vi "Render Inverted Section with Empty Map Object Array.vi"(8 "Error In":errorcluster) -> (0 "Error Out":errorcluster)   [LabVIEW 2018, in "Tests.lvlib" / "Render.lvlib"]
uses:
  Render.lvlib
  <vilib>/addons/_JKI Toolkits/Caraya/classes/Test/Test.lvclass
  <vilib>/addons/_JKI Toolkits/Caraya/classes/Assert/Assert.lvclass
  src/Toolkit/Data/Array/Array.lvclass
  src/Toolkit/Low-Level/Renderer/Abstract/Render to String.vi
  src/Toolkit/Low-Level/Support/Lex String.vi
  src/Toolkit/Data/Array/Support/From Data.vi
  src/Toolkit/Data/Pair/Pair.lvclass
  src/Toolkit/Data/Pair/Support/From Datum.vi
  src/Toolkit/Data/Map/Map.lvclass
  src/Toolkit/Low-Level/Context/Compiler.lvclass
  D:/Users/cfield/Code/Field R&D Services/Labstache/src/Toolkit/Data/Datum/Datum.lvclass
  src/Toolkit/Low-Level/Nodes/Root/Root.lvclass
  D:/Users/cfield/Code/Field R&D Services/Labstache/src/Toolkit/Low-Level/Nodes/NonTerminal/NonTerminal.lvclass
  D:/Users/cfield/Code/Field R&D Services/Labstache/src/Toolkit/Low-Level/Nodes/Node/Node.lvclass
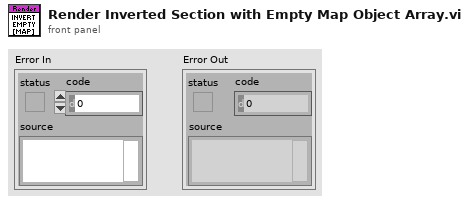
[diagram p1: front panel]
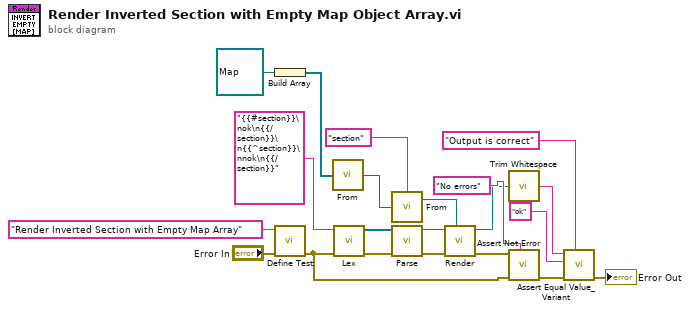
[diagram p0: block diagram]
diagram:
  n1 = Build Array(refnum<class "Map.lvclass"> refnum ("Toolkit.lvlib:Data.lvlib:Map.lvclass")) -> (w1:refnum<class "Map.lvclass">[])
  n2 = call <vilib>:"Define Test.vi"("error in (no error)"="Error In", "Label (VI Title)"="Render Inverted Section with Empty Map Array") -> ("error out"=w11:errorcluster)  [unwired: 9 in]
  n3 = call-poly "From.vi"("Data"=w1) -> ("Array"=w4:refnum<class "Array.lvclass">)  [unwired: 1 in]
  n4 = call-poly "Lex.vi"("Error In"=w11, "Input"="{{#section}}\nok\n{{/section}}\n{{^section}}\nnok\n{{/section}}") -> ("Error Out"=w12:errorcluster, "Tokens"=w13:refnum<class "Token.lvclass">[])  [unwired: 8 in]
  n5 = call-poly "From.vi"("Value"=w4, "Key"="section") -> ("Pair"=w3:refnum<class "Pair.lvclass">)
  n6 = call "Parse.vi"("Error In"=w12, "Tokens"=w13) -> ("Error Out"=w14:errorcluster, "Abstract Syntax Tree"=w10:refnum<class "Root.lvclass">)  [unwired: 8 in]
  n7 = call-poly "Render.vi"(7:w3, "Error In"=w14, "Context In"=w10) -> ("Error Out"=w15:errorcluster, "Context Out"=w7:refnum<class "Compiler.lvclass">)  [unwired: 6 in, 1 out]
  n8 = call <vilib>:"Trim Whitespace.vi"("string"=w7) -> ("trimmed string"=w6:string)  [unwired: 1 in]
  n9 = call <vilib>:"Assert Not Error.vi"("Label"="No errors", "error in (no error)"=w11, "Not Error?"=w15) -> ("error out"=w18:errorcluster)  [unwired: 8 in]
  n10 = call <vilib>:"Assert Equal Value_Variant.vi"("Label"="Output is correct", "error in (no error)"=w18, "Y"="ok", "X"=w6) -> ("error out"=→"Error Out":errorcluster)  [unwired: 7 in]
